vi "Read Cluster.vi"(8 "error in":errorcluster, 10 "Type in":variant, 11 "config-base in":refnum<class "config-base.lvclass">) -> (0 "error out":errorcluster, 2 "Value Cluster out":variant, 3 "config-base out":refnum<class "config-base.lvclass">)   [LabVIEW 2022 SP3, in "hse-config.lvlib" / "config-base.lvclass"]
doc: "Returns a cluster of config values (can be nested) of the same type as \"Type in\".\nUse the \"Variant to Data\" function to convert the Variant back to the cluster type.\n\n____\nHAMPEL SOFTWARE ENGINEERING v3.8.0 (2023-12-18 14:41)"
uses:
  config-base.lvclass
  config-base.lvclass/config-base.ctl
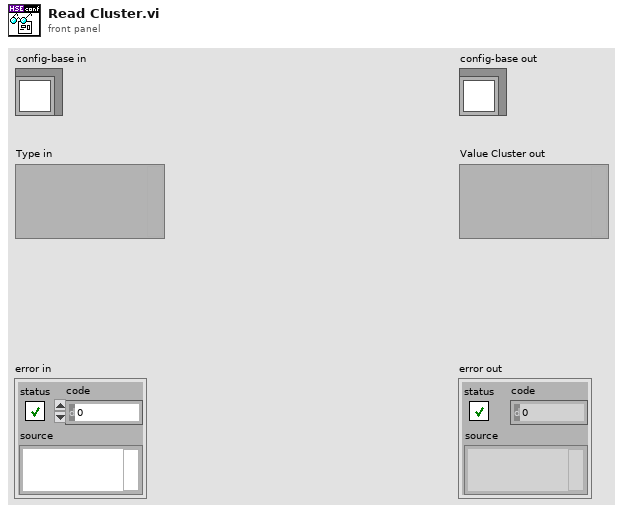
[diagram p1: front panel]
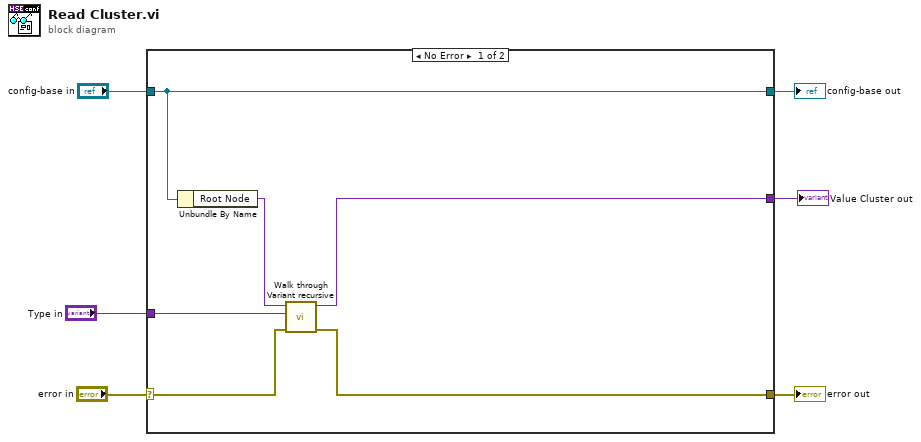
[diagram p0: block diagram]
diagram:
  n1 = case shown="No Error" "error in" {
    selector: "error in" -> [w12 w14]
    tunnel: [w8 w14] -> w5
    tunnel: [w10 w13] -> w3
    tunnel: "config-base in" -> [w10 w13]
    tunnel: "Type in" -> [w11 _]
    tunnel: [w7 _] -> w1
    frame No Error {
      n2 = Unbundle By Name(w10) -> ("Root Node"=w9:variant)
      n3 = call "Walk through Variant recursive.vi"("error in"=w12, "Type in"=w11, "Node in"=w9) -> ("error out"=w8:errorcluster, "Node out"=w7:variant)  [unwired: 7 in]
    }
    frame Error {
    }
  }
  "error out" <- w5
  "config-base out" <- w3
  "Value Cluster out" <- w1
